vi "Create Document.vi"(8 "error in (no error)":errorcluster, 10 "Root Element Name":string="testsuites") -> (0 "error out":errorcluster, 2 "Root Element":refnum<k20>, 3 "Document":refnum<k20>)   [LabVIEW 2013, in "XML.lvlib"]
doc: "Creates a new document with the specified root element. The caller is responsible for cleaning up references."
uses:
  XML.lvlib
  <vilib>/xml/NI_XML.lvlib
  <resource>/objmgr/DOMUserDefRef.rc
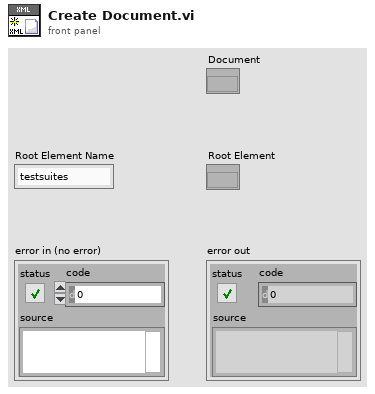
[diagram p1: front panel]
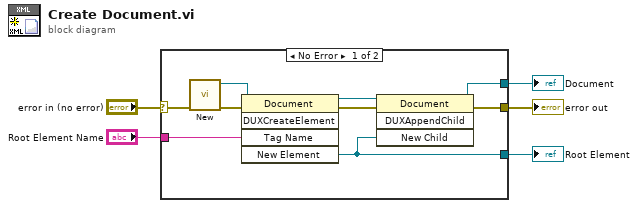
[diagram p0: block diagram]
diagram:
  n1 = case shown="No Error" "error in (no error)" {
    selector: "error in (no error)" -> [w6 w15]
    tunnel: "Root Element Name" -> [w12 _]
    tunnel: [w10 _] -> w4
    tunnel: [w8 w15] -> w3
    tunnel: [w7 _] -> w2
    frame No Error {
      n2 = call <vilib>:"New.vi"("error in (no error)"=w6) -> ("error out"=w14:errorcluster, "DOM document out"=w9:refnum<k20>)  [unwired: 7 in]
      n3 = invoke class="Document" method="DUXCreateElement"(reference=w9, error in=w14, "Tag Name"=w12) -> (reference out=w11:refnum<k20>, error out=w13:errorcluster, "New Element"=w10:refnum<k20>)  [unwired: 2 in, 2 out]
      n4 = invoke class="Document" method="DUXAppendChild"(reference=w11, error in=w13, "New Child"=w10) -> (reference out=w7:refnum<k20>, error out=w8:errorcluster)  [unwired: 1 in, 2 out]
    }
    frame Error {
    }
  }
  "error out" <- w3
  "Document" <- w2
  "Root Element" <- w4
